vi "ke37xx Configure Blender Mode.vi"(0 "VISA Resource Name":refnum<visa-resource-name>, 5 "Blender (1)":u8=1 min=1 max=2, 7 "Mode (0: AND)":enum16{"AND Mode", "OR Mode"}(ring), 11 "error in (no error)":errorcluster) -> (4 "VISA Resource Name Out":refnum<visa-resource-name>, 15 "error out":errorcluster)   [LabVIEW 2009, in "Keithley 3700 Series.lvlib"]
doc: "This VI allows you to configure themode in which the blender operates. In OR-mode, the blender enters the detected state when any one of its stimulus inputs becomes true. In AND-mode, the blender waits for all of its stimulus inputs to be true before it enters the detected state."
uses:
  <instrlib>/Keithley 3706/Keithley 3700 Series.lvlib
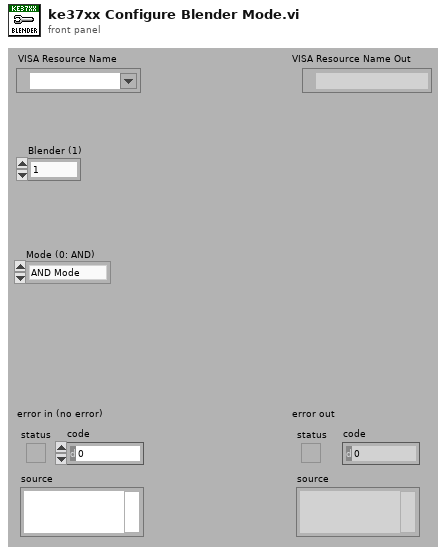
[diagram p1: front panel]
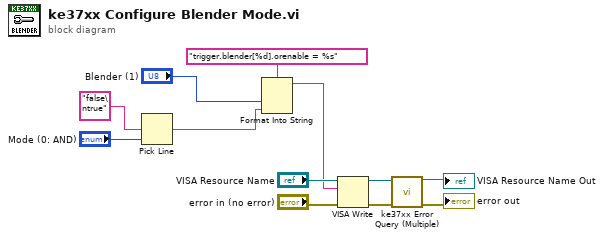
[diagram p0: block diagram]
diagram:
  n1 = Pick Line(multi-line string="false\ntrue", line index="Mode (0: AND)") -> (output string=w1:string)  [unwired: 1 out]
  n2 = Format Into String(format string="trigger.blender[%d].orenable = %s" ("multi-line string"), "Blender (1)", w1) -> (resulting string=w6:string)  [unwired: 2 in, 1 out]
  n3 = VISA Write(VISA resource name="VISA Resource Name", write buffer=w6, error in (no error)="error in (no error)") -> (VISA resource name out=w8:refnum<visa-resource-name>, error out=w7:errorcluster)  [unwired: 1 out]
  n4 = call <instrlib>:"ke37xx Error Query (Multiple).vi"("VISA resource name"=w8, "error in (no error)"=w7) -> ("VISA resource name out"=→"VISA Resource Name Out":refnum<visa-resource-name>, "error out"=→"error out":errorcluster)  [unwired: 12 out]
